vi "viewvi.vi"(6 "item tag":string, 7 "menu reference":refnum<k9>) -> (0 "error out":errorcluster)   [LabVIEW 2010]
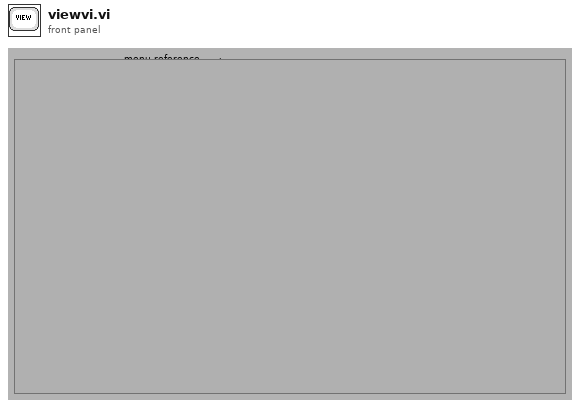
[diagram p1: front panel]
types:
  T1 = enum32{"invalid VI type", "Standard VI", "Control VI", "Global VI", "Polymorphic VI", "Configuration VI", "SubSystem", "Facade VI", "Method VI", "Statechart Diagram VI"}
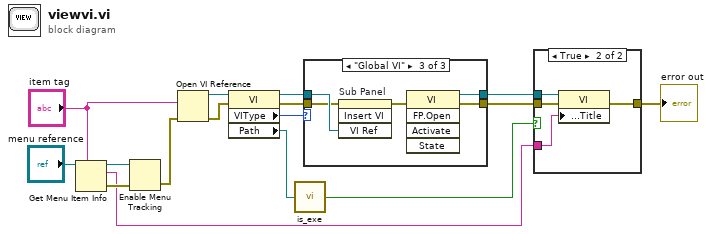
[diagram p0: block diagram]
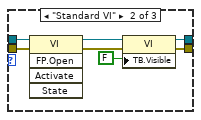
[diagram p4: hidden frame]
diagram:
  n1 = Get Menu Item Info(7:"item tag", 11:"menu reference") -> (0:w13:errorcluster, 2:w4:string, 3:w16:refnum<k9>)  [unwired: 1 in, 4 out]
  n2 = Enable Menu Tracking(2:w13, 4:w16) -> (0:w12:errorcluster)  [unwired: 1 in, 1 out]
  n3 = Open VI Reference(vi path="item tag", error in (no error)=w12) -> (vi reference=w14:refnum<vi>, error out=w10:errorcluster)  [unwired: 4 in]
  n4 = property class="VI"(reference=w14, error in=w10) -> (reference out=w8:refnum<vi>, error out=w7:errorcluster, "VIType"=w9:T1, "Path"=w6:path)
  n5 = call "is_exe.vi"("path"=w6) -> ("exe?"=w2:bool)  [unwired: 2 in, 2 out]
  n6 = case shown="\"Global VI\"" w9 {
    tunnel: [_ w20 w26] -> w3
    tunnel: w8 -> [_ w19 w28]
    tunnel: w7 -> [_ w18 w24]
    tunnel: [_ w17 w25] -> w5
    frame "invalid VI type", Default {
    }
    frame "Standard VI" {
      n7 = invoke class="VI" method="FP.Open"(reference=w19, error in=w18) -> (reference out=w22:refnum<vi>, error out=w23:errorcluster)  [unwired: 3 in, 3 out]
      n8 = property class="VI"(reference=w22, error in=w23, "TB.Visible"=FALSE ("Tool Bar:Visible")) -> (reference out=w17:refnum<vi>, error out=w20:errorcluster)
    }
    frame "Global VI" {
      n9 = invoke on="Sub Panel" class="SubPanel" method="Insert VI"(error in=w24, "VI Ref"=w28) -> (error out=w27:errorcluster)  [unwired: 2 in, 3 out]
      n10 = invoke class="VI" method="FP.Open"(error in=w27) -> (reference out=w25:refnum<vi>, error out=w26:errorcluster)  [unwired: 4 in, 3 out]
    }
  }
  n11 = case shown="True" w2 {
    tunnel: w5 -> [_ w33]
    tunnel: w4 -> [_ w32]
    tunnel: w3 -> [w29 w31]
    tunnel: [w29 w30] -> w1
    frame False {
    }
    frame True {
      n12 = property class="VI"(reference=w33, error in=w31, "Front Panel.Title"=w32) -> (error out=w30:errorcluster)  [unwired: 1 out]
    }
  }
  "error out" <- w1
